vi "Query Bias Level.vi"(8 "error in (no error)":errorcluster, 9 "Channel List (\"\")":string, 11 "VISA resource name":refnum<visa-resource-name>) -> (0 "error out":errorcluster, 2 "Bias Level (0)":dbl, 3 "VISA resource name out":refnum<visa-resource-name>)   [LabVIEW 2016, in "Keithley DMM6500 DAQ6500 Series.lvlib"]
doc: "Queries the amount of current the instrument is sourcing when it makes measurements."
uses:
  Keithley DMM6500 DAQ6500 Series.lvlib
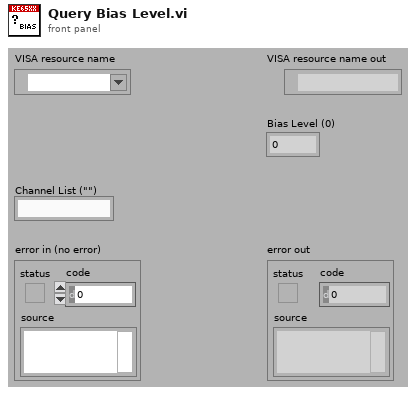
[diagram p1: front panel]
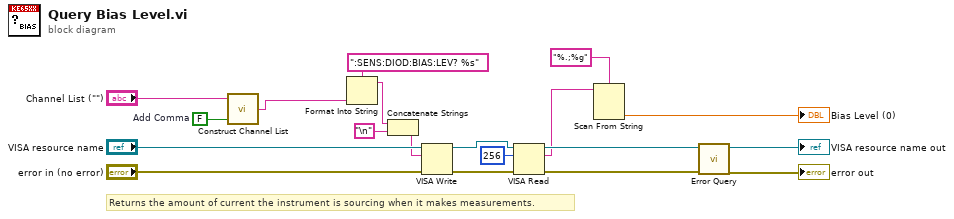
[diagram p0: block diagram]
diagram:
  w5 = FALSE  # Add Comma
  # "Returns the amount of current the instrument is sourcing when it makes measurements."
  n1 = call "Construct Channel List.vi"("Add Comma (True)"=w5, "Channel List"="Channel List (\"\")") -> ("Channel List String"=w1:string)  [unwired: 1 in]
  n2 = Format Into String(format string=":SENS:DIOD:BIAS:LEV? %s", w1) -> (resulting string=w3:string)  [unwired: 2 in, 1 out]
  n3 = Concatenate Strings(w3, "\n") -> (w4:string)
  n4 = VISA Write(VISA resource name="VISA resource name", write buffer=w4, error in (no error)="error in (no error)") -> (VISA resource name out=w10:refnum<visa-resource-name>, error out=w14:errorcluster)  [unwired: 1 out]
  n5 = VISA Read(VISA resource name=w10, byte count=u32 256, error in (no error)=w14) -> (VISA resource name out=w9:refnum<visa-resource-name>, read buffer=w8:string, error out=w13:errorcluster)  [unwired: 1 out]
  n6 = Scan From String(format string="%.;%g", input string=w8) -> (output 1=→"Bias Level (0)":dbl)  [unwired: 3 in, 3 out]
  n7 = call "Error Query.vi"("error in (no error)"=w13, "VISA resource name"=w9) -> ("error out"=→"error out":errorcluster, "VISA resource name out"=→"VISA resource name out":refnum<visa-resource-name>)  [unwired: 6 in, 2 out]
